vi "舵机main(子VI).vi"(6 "error in (no error)":errorcluster, 10 "null offset":bool, 11 "舵机":dbl(slide) min=-100.0 max=100.0 scale=-200.0..200.0) -> (4 "error out":errorcluster)   [LabVIEW 2014]
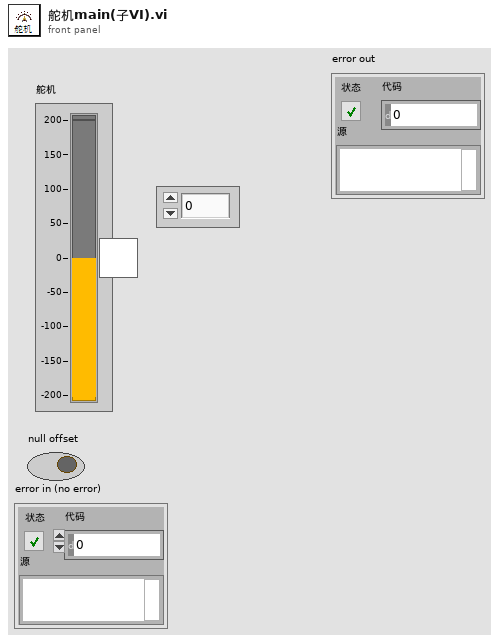
[diagram p1: front panel]
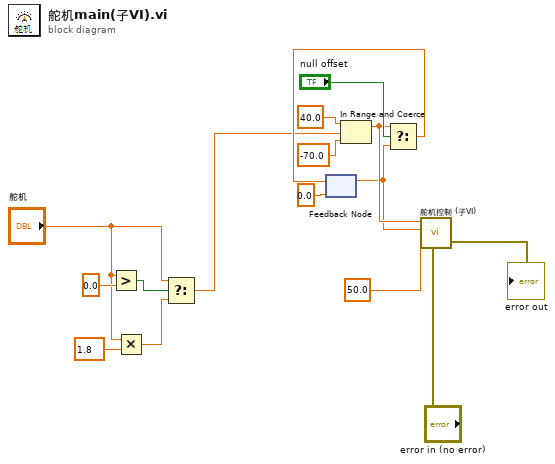
[diagram p0: block diagram]
diagram:
  n1 = Greater?(x="舵机", y=0.0) -> (0:w6:bool)
  n2 = Multiply(x="舵机", y=1.8) -> (x*y=w1:dbl)
  n3 = Select(t="舵机", s=w6, f=w1) -> (s? t:f=w4:dbl)
  n4 = feedback #1(0.0 ("position [%FS]")) -> (w11:dbl)
  n5 = In Range and Coerce(upper limit=40.0 ("上限"), x=w4, lower limit=-70.0 ("下限")) -> (coerced(x)=w15:dbl)  [unwired: 1 out]
  n6 = Select(t=w15, s="null offset", f=w11) -> (s? t:f=w12:dbl)
  n7 = feedback-in #1(w12) -> ()
  n8 = call "舵机控制 (子VI).vi"("error in (no error)"="error in (no error)", "freq [Hz]"=50.0, "position [%FS]"=w11, "上限"=w15) -> ("error out"=→"error out":errorcluster)  [unwired: 5 in, 2 out]
